vi "bazowy_TN_inz.vi"() -> ()   [LabVIEW 2019]
panel:
  out "komTESTz":bool
  out "komTESTdo":bool
  out "Objętość - zb4":dbl
  out "Objętość - zb3":dbl
  out "Objętość - zb2":dbl
  out "Objętość - zb1":dbl
  out "Zawór spustowy Z4":bool
  out "Zawór spustowy Z3":bool
  out "Zawór spustowy Z2":bool
  out "Zawór spustowy Z1":bool
  out "P8 - konserwacja":bool
  out "P7 - konserwacja":bool
  out "P6 - konserwacja":bool
  out "P5 - konserwacja":bool
  out "P4 - konserwacja":bool
  out "P3 - konserwacja":bool
  out "P2 - konserwacja":bool
  out "P1 - konserwacja":bool
  out "Awaryjne zatrzymanie pomp i opróżnienie  zbiorników (Awaria)":bool
  out "Czas utrzymania temperatury - zb4":u32
  out "Temperatura maksymalna - zb4":sgl
  out "Objętość cieczy - zb4":sgl
  out "Czas utrzymania temperatury - zb3":u32
  out "Temperatura maksymalna - zb3":sgl
  out "Objętość cieczy - zb3":sgl
  out "Czas utrzymania temperatury - zb2":u32
  out "Temperatura maksymalna - zb2":sgl
  out "Czas utrzymania temperatury - zb1":u32
  out "Objętość cieczy - zb2":sgl
  out "Temperatura maksymalna - zb1":sgl
  out "Objętość cieczy - zb1":sgl
  out "Grzałka 4":bool
  out "Grzałka 3":bool
  out "Grzałka 2":bool
  out "Grzałka 1":bool
  out "Pompa 8":bool
  out "Pompa 7":bool
  out "Pompa 6":bool
  out "Pompa 5":bool
  out "Pompa 4":bool
  out "Pompa 3":bool
  out "Pompa 2":bool
  out "Zawór wlotowy 3":bool
  out "Zawór wlotowy 2":bool
  out "Temp cieczy w zb 4":sgl
  out "Temp cieczy w zb 3":sgl
  out "Temp cieczy w zb 2":sgl
  out "Temp cieczy w zb 1":sgl
  out "Temp P8":sgl
  out "Temp P7":sgl
  out "Temp P6":sgl
  out "Temp P5":sgl
  out "Temp P4":sgl
  out "Temp P3":sgl
  out "Temp P2":sgl
  out "Temp P1":sgl=20.009169
  out "Pompa 1":bool
  out "Zawór wlotowy 1":bool
  out "Inf - temp przed zb3":dbl
  out "Inf - temp przed zb2":dbl
  out "Inf - temp przed zb1":dbl
  out "Inf - temp przed zb4":dbl
  out "Inf - poz przed zb3":dbl
  out "Inf - poz przed zb2":dbl
  out "Inf - poz przed zb1":dbl
  out "Temp. cieczy w zb 4":sgl
  out "Temp i objętość cieczy w zb 4":cluster{sgl, "T":dbl}(graph)
  out "Zbiornik 4":sgl(slide) scale=0.0..300.0
  out "Zbiornik 3":sgl(slide) scale=0.0..100.0
  out "Zbiornik 2":sgl(slide) scale=0.0..100.0
  out "Zbiornik 1":sgl(slide) scale=0.0..100.0
  out "Temp. cieczy w zb 3":sgl
  out "Temp. cieczy w zb 2":sgl
  out "Temp. cieczy w zb 1":sgl
  out "Temp i objętość cieczy w zb 3":cluster{"Zbiornik 3":sgl, "T":dbl}(graph)
  out "Temp i objętość cieczy w zb 2":cluster{"Zbiornik 2":sgl, "T":dbl}(graph)
  out "Temp i objętość cieczy w zb 1":cluster{"Zbiornik 1":sgl, "T":dbl}(graph)
  in  "r4d":sgl=0.002
  in  "r4":sgl=0.9977
  in  "r3d":sgl=0.02
  in  "r3":sgl=0.968
  in  "Tk":sgl=100.0
  in  "Tot":sgl=20.0
  out "Temp. P8":sgl
  out "Temp. P7":sgl
  out "temp P7 - P8":cluster{"T":dbl, "T":dbl, sgl}(graph)
  out "Temp. P6":sgl
  out "Temp. P5":sgl
  out "temp P5 - P6":cluster{"T":dbl, "T":dbl, "Zbiornik 3":sgl}(graph)
  out "Temp. P4":sgl
  out "Temp. P3":sgl
  out "temp P3 - P4":cluster{"T":dbl, "T":dbl, "Zbiornik 2":sgl}(graph)
  out "Temp. P2":sgl
  out "Temp. P1":sgl
  out "temp P1 - P2":cluster{"T":dbl, "T":dbl, "Zbiornik 1":sgl}(graph)
  in  "To":sgl=20.0
  in  "Ts":sgl=80.0
  in  "r2":sgl=0.92
  in  "r1":sgl=0.92
  in  "stop":bool
  # "Temperatura pomp"
  # "460 na wykres"
  # "(°C)"
  # "(°C)"
  # "(°C)"
  # "(°C)"
  # "(°C)"
  # "(°C)"
  # "(°C)"
  # "(°C)"
  # "(°C)"
  # "(°C)"
  # "Temperatura i objętość cieczy w zbiornikach 1, 2, 3 i 4"
  # "(°C)"
  # "(°C)"
  # "Nastawy grzanie"
  # "Nastawy chłodzenie"
  # "(°C)"
  # "(l)"
  # "(l)"
  # "(°C)"
  # "(°C)"
  # "(l)"
  # "(l)"
  # "(°C)"
  # "Nie do odczytu. Wartości chwilowe dla wyliczenia temperatury cieczy z zbiorników po zmieszaniu się"
  # "Parametry zadane w aktualnym procesie (partii produktu)"
  # "Zbiornik 1"
  # "Zbiornik 2"
  # "Zbiornik 3"
  # "(°C)"
  # "(°C)"
  # "(°C)"
  # "Zbiornik 4"
  # "(°C)"
  # "(°C)"
  # "(°C)"
  # "(°C)"
  # "(°C)"
  # "(°C)"
  # "(°C)"
  # "(°C)"
  # "(°C)"
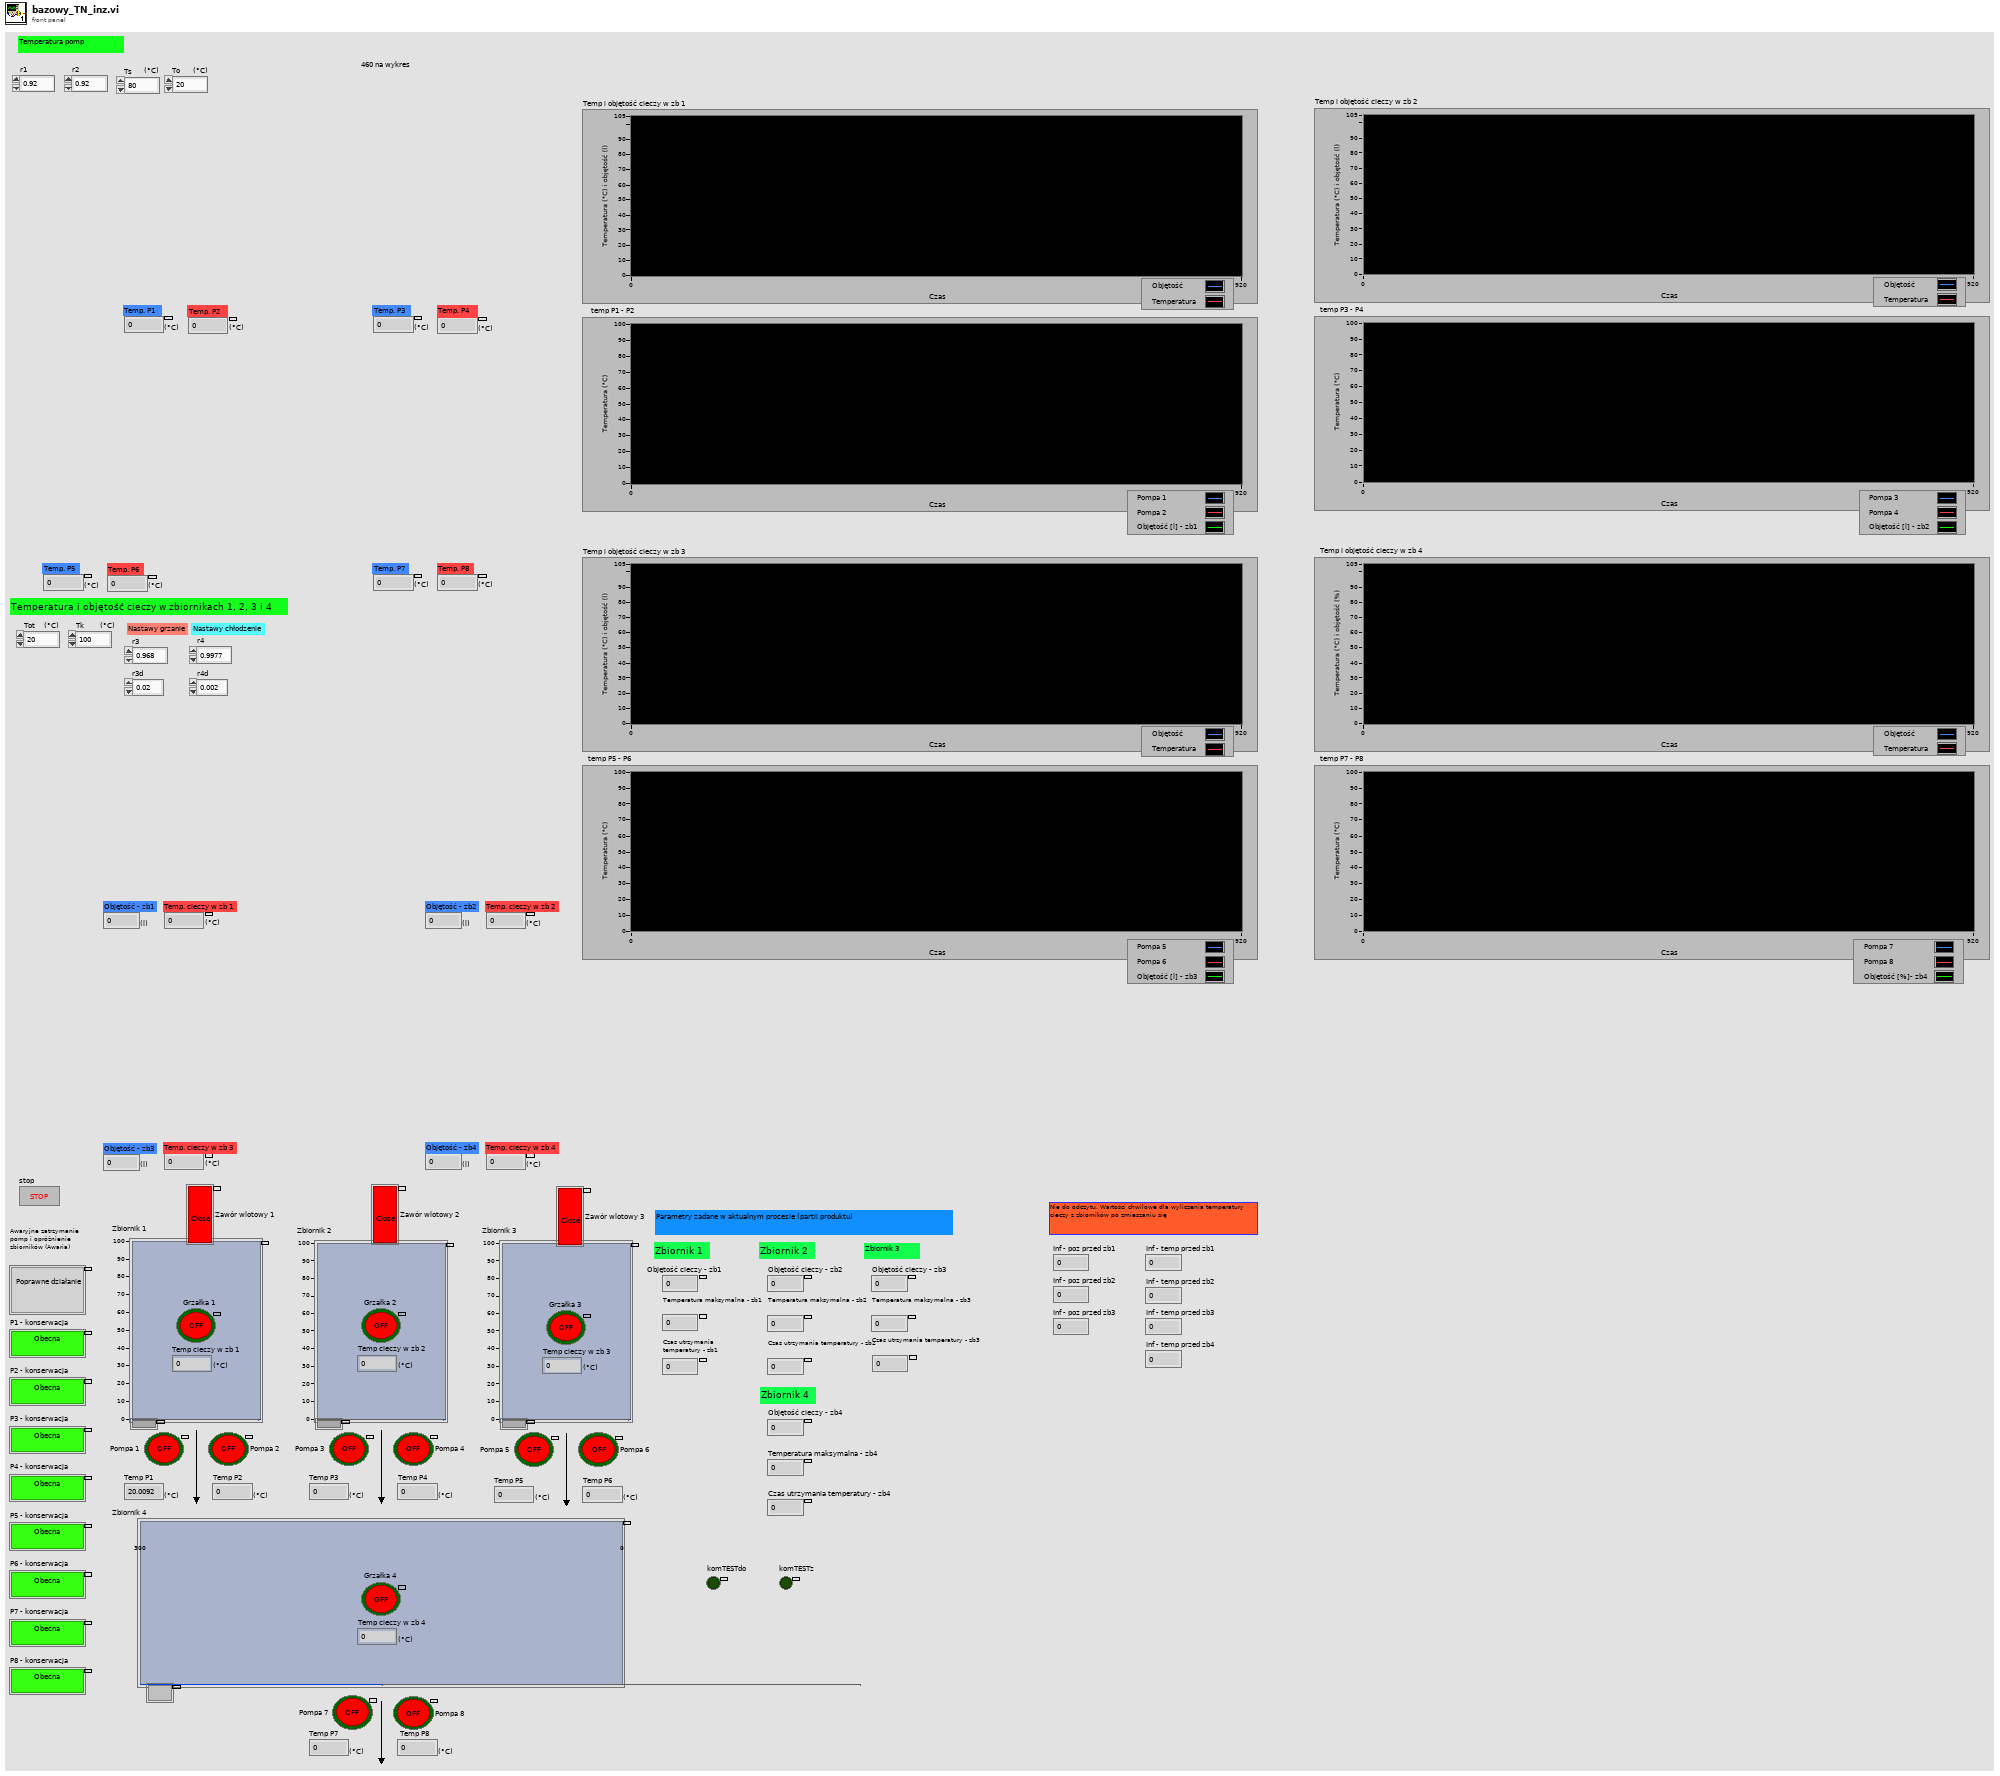
[diagram p1: front panel]
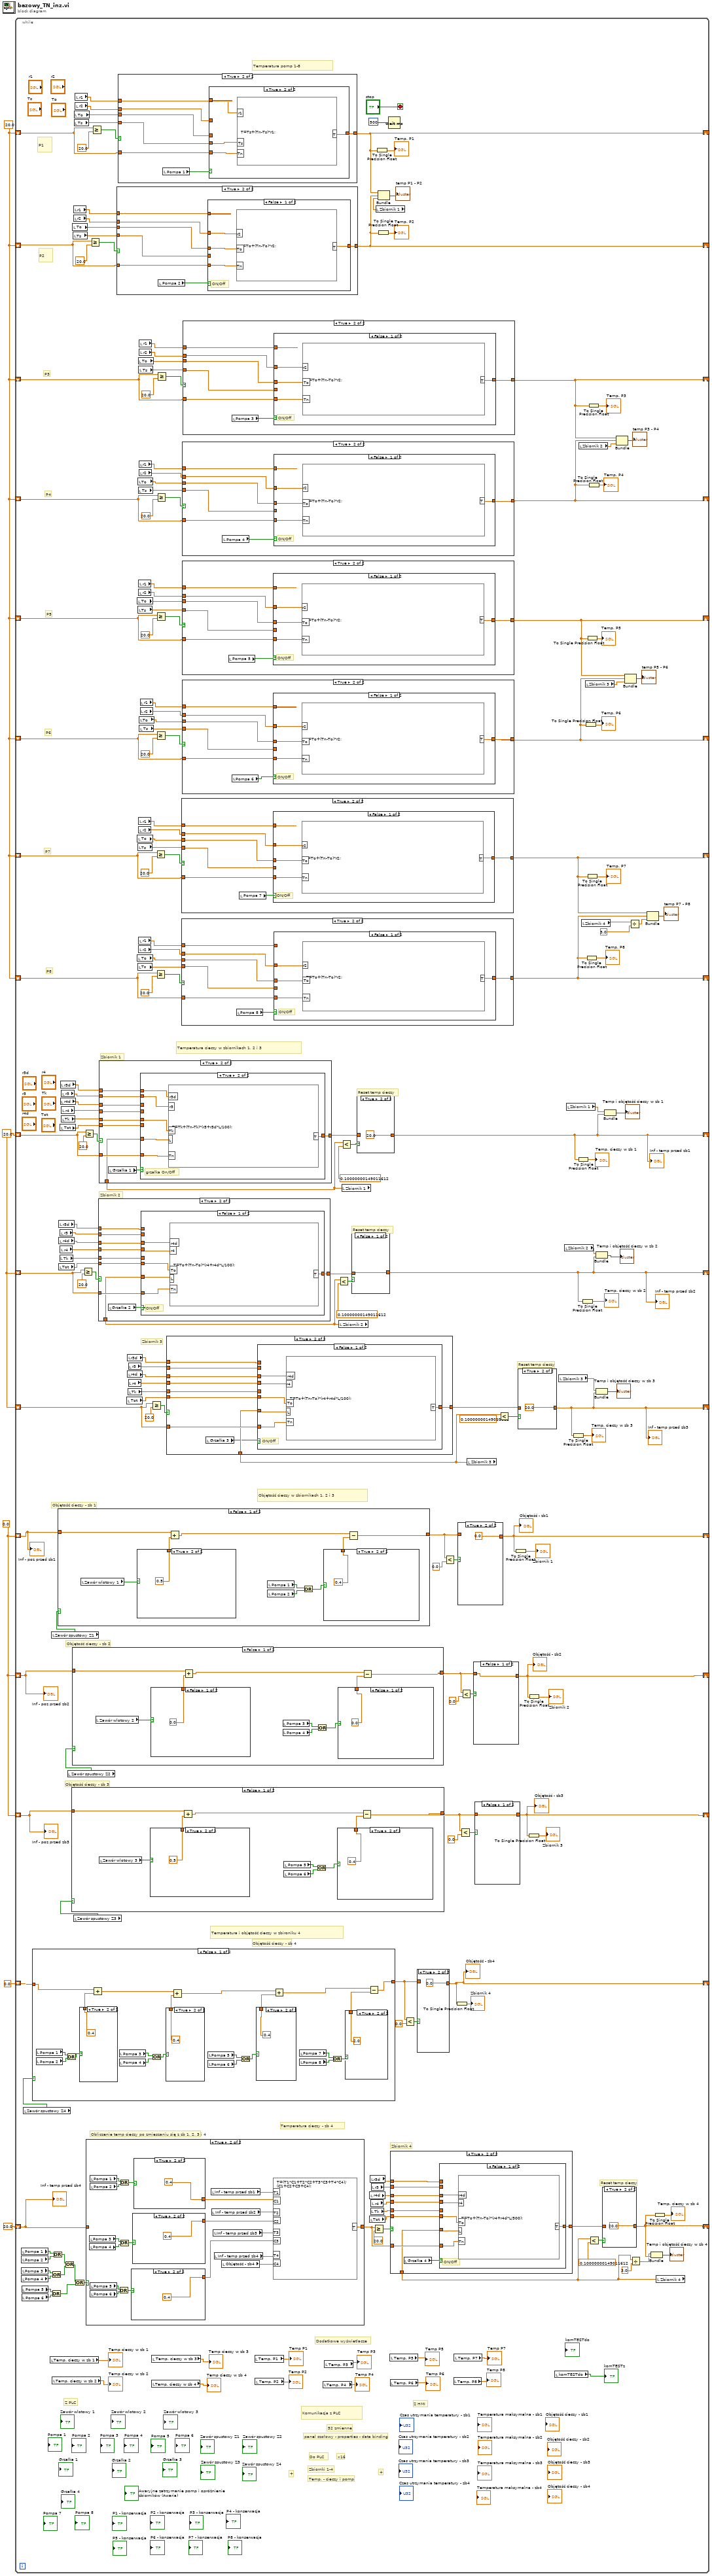
[diagram p0: block diagram]
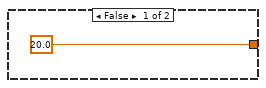
[diagram p2: hidden frame]
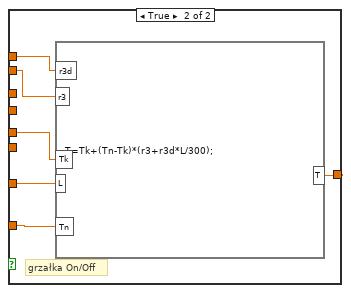
[diagram p3: hidden frame]
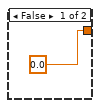
[diagram p5: hidden frame]
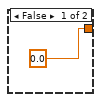
[diagram p6: hidden frame]
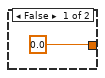
[diagram p7: hidden frame]
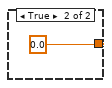
[diagram p9: hidden frame]
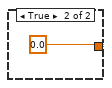
[diagram p10: hidden frame]
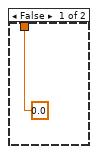
[diagram p12: hidden frame]
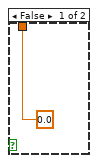
[diagram p13: hidden frame]
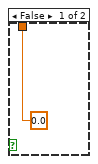
[diagram p14: hidden frame]
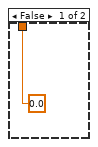
[diagram p15: hidden frame]
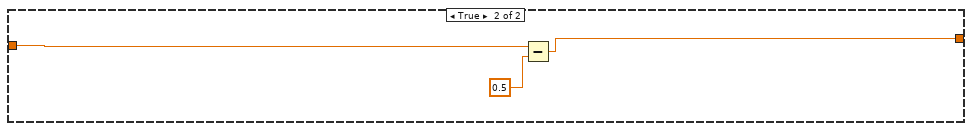
[diagram p16: hidden frame]
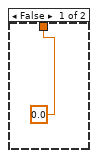
[diagram p18: hidden frame]
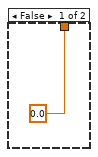
[diagram p19: hidden frame]
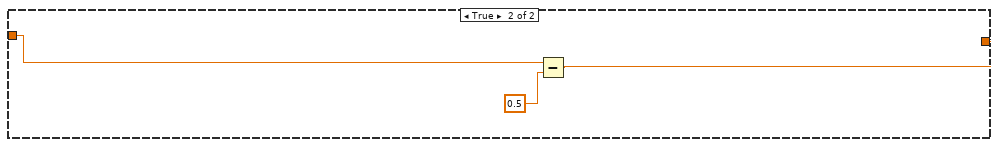
[diagram p20: hidden frame]
diagram:
  w4 = 0.0
  w1 = 20.0
  w5 = 20.0
  n1 = while {
    shift-right: [w60] -> _
    shift-left: w5 -> [w207]
    shift-right: [w59] -> _
    shift-left: w5 -> [w204]
    shift-right: [w58] -> _
    shift-left: w5 -> [w201]
    shift-right: [w57] -> _
    shift-left: w5 -> [w190]
    shift-right: [w53] -> _
    shift-left: w5 -> [w189]
    shift-right: [w55] -> _
    shift-left: w5 -> [w188]
    shift-right: [w52] -> _
    shift-left: w5 -> [w187]
    shift-right: [w54] -> _
    shift-left: w5 -> [w186]
    shift-right: [w16] -> _
    shift-left: w1 -> [w21]
    shift-right: [w15] -> _
    shift-left: w1 -> [w83]
    shift-right: [w14] -> _
    shift-left: w1 -> [w22]
    shift-right: [w37] -> _
    shift-left: w4 -> [w13]
    shift-right: [w39] -> _
    shift-left: w4 -> [w23]
    shift-right: [w38] -> _
    shift-left: w4 -> [w79]
    shift-right: [w41] -> _
    shift-left: 20.0 -> [w25]
    shift-right: [w40] -> _
    shift-left: 0.0 -> [w24]
    stop <- "stop" stop-if-true
    # "Temperatura cieczy - zb 4"
    # "x16"
    # "52 zmienne"
    # "Do PLC"
    # "Z PLC"
    # "Z HMI"
    # "panel czołowy - properties - data binding"
    # "Temp. - cieczy i pomp"
    # "Zbiornki 1-4"
    # "+"
    # "+"
    # "Dodatkowe wyświetlacze"
    # "Komunikacja z PLC"
    # "Obliczenie temp cieczy po zmieszaniu się z zb 1, 2, 3 i 4"
    # "Zbiornik 4"
    # "Reset temp cieczy"
    # "Objętość cieczy - zb 4"
    # "Temperatura i objętość cieczy w zbironiku 4"
    # "Objętość cieczy - zb 3"
    # "Objętość cieczy - zb 2"
    # "Objętość cieczy - zb 1"
    # "Objętość cieczy w zbiornikach 1, 2 i 3"
    # "Zbiornik 3"
    # "Reset temp cieczy"
    # "Zbiornik 2"
    # "Reset temp cieczy"
    # "Zbiornik 1"
    # "Reset temp cieczy"
    # "P8"
    # "P7"
    # "P6"
    # "P5"
    # "P4"
    # "Temperatura cieczy w zbiornikach 1, 2 i 3"
    # "P3"
    # "P2"
    # "P1"
    # "Temperatura pomp 1-8"
    n2 = local read "Pompa 1"() -> (w36:bool)
    n3 = local read "Pompa 2"() -> (w35:bool)
    n4 = local read "Pompa 3"() -> (w34:bool)
    n5 = local read "Pompa 4"() -> (w33:bool)
    n6 = local read "Pompa 5"() -> (w32:bool)
    n7 = local read "Pompa 6"() -> (w31:bool)
    n8 = local read "Zawór spustowy Z4"() -> (w95:bool)
    n9 = case shown="False" w95 {
      tunnel: [w284 w297] -> w118
      tunnel: w24 -> [w288 w298]
      frame False {
        n10 = local read "Pompa 1"() -> (w275:bool)
        n11 = local read "Pompa 2"() -> (w274:bool)
        n12 = Or(x=w275, y=w274) -> (x .or. y?=w280:bool)
        n13 = case shown="True" w280 {
          tunnel: [0.0 0.4] -> w279
          frame False {
          }
          frame True {
          }
        }
        n14 = Add(x=w288, y=w279) -> (x+y=w287:dbl)
        n15 = local read "Pompa 3"() -> (w273:bool)
        n16 = local read "Pompa 4"() -> (w272:bool)
        n17 = Or(x=w273, y=w272) -> (x .or. y?=w281:bool)
        n18 = case shown="True" w281 {
          tunnel: [0.0 0.4] -> w278
          frame False {
          }
          frame True {
          }
        }
        n19 = Add(x=w287, y=w278) -> (x+y=w286:dbl)
        n20 = local read "Pompa 5"() -> (w271:bool)
        n21 = local read "Pompa 6"() -> (w270:bool)
        n22 = Or(x=w271, y=w270) -> (x .or. y?=w282:bool)
        n23 = case shown="True" w282 {
          tunnel: [0.0 0.4] -> w277
          frame False {
          }
          frame True {
          }
        }
        n24 = Add(x=w286, y=w277) -> (x+y=w285:dbl)
        n25 = local read "Pompa 7"() -> (w269:bool)
        n26 = local read "Pompa 8"() -> (w268:bool)
        n27 = Or(x=w269, y=w268) -> (x .or. y?=w283:bool)
        n28 = case shown="True" w283 {
          tunnel: [0.0 2.0] -> w276
          frame False {
          }
          frame True {
          }
        }
        n29 = Subtract(x=w285, y=w276) -> (x-y=w284:dbl)
      }
      frame True {
        n30 = Subtract(x=w298, y=0.5) -> (x-y=w297:dbl)
      }
    }
    n31 = local read "Temp. cieczy w zb 1"() -> (→"Temp cieczy w zb 1":sgl)
    n32 = Or(x=w32, y=w31) -> (x .or. y?=w28:bool)
    n33 = Or(x=w34, y=w33) -> (x .or. y?=w29:bool)
    n34 = local read "Zawór spustowy Z1"() -> (w93:bool)
    n35 = Or(x=w36, y=w35) -> (x .or. y?=w30:bool)
    n36 = local read "Temp. cieczy w zb 2"() -> (→"Temp cieczy w zb 2":sgl)
    n37 = case shown="False" w93 {
      tunnel: w13 -> [w342 w349]
      tunnel: [w340 w347] -> w127
      frame False {
        n38 = local read "Zawór wlotowy 1"() -> (w336:bool)
        n39 = case shown="True" w336 {
          tunnel: [0.0 0.5] -> w338
          frame False {
          }
          frame True {
          }
        }
        n40 = Add(x=w342, y=w338) -> (x+y=w341:dbl)
        n41 = local read "Pompa 1"() -> (w335:bool)
        n42 = local read "Pompa 2"() -> (w334:bool)
        n43 = Or(x=w335, y=w334) -> (x .or. y?=w339:bool)
        n44 = case shown="True" w339 {
          tunnel: [0.0 0.4] -> w337
          frame False {
          }
          frame True {
          }
        }
        n45 = Subtract(x=w341, y=w337) -> (x-y=w340:dbl)
      }
      frame True {
        n46 = Subtract(x=w349, y=0.5) -> (x-y=w347:dbl)
      }
    }
    n47 = local read "Tot"() -> (w136:sgl)
    n48 = local read "r3d"() -> (w141:sgl)
    n49 = local read "r4d"() -> (w139:sgl)
    n50 = local read "Tk"() -> (w137:sgl)
    n51 = local read "Tot"() -> (w142:sgl)
    n52 = local read "r3"() -> (w140:sgl)
    n53 = local read "r4"() -> (w138:sgl)
    n54 = local read "r3d"() -> (w147:sgl)
    n55 = local read "r4d"() -> (w145:sgl)
    n56 = local read "Tk"() -> (w143:sgl)
    n57 = local read "r3"() -> (w146:sgl)
    n58 = local read "r4"() -> (w144:sgl)
    n59 = Or(x=w30, y=w29) -> (x .or. y?=w27:bool)
    n60 = local read "Zawór spustowy Z2"() -> (w92:bool)
    n61 = case shown="False" w92 {
      tunnel: w79 -> [w326 w333]
      tunnel: [w324 w331] -> w121
      frame False {
        n62 = local read "Zawór wlotowy 2"() -> (w320:bool)
        n63 = case shown="False" w320 {
          tunnel: [0.0 0.5] -> w322
          frame False {
          }
          frame True {
          }
        }
        n64 = Add(x=w326, y=w322) -> (x+y=w325:dbl)
        n65 = local read "Pompa 3"() -> (w319:bool)
        n66 = local read "Pompa 4"() -> (w318:bool)
        n67 = Or(x=w319, y=w318) -> (x .or. y?=w323:bool)
        n68 = case shown="False" w323 {
          tunnel: [0.0 0.4] -> w321
          frame False {
          }
          frame True {
          }
        }
        n69 = Subtract(x=w325, y=w321) -> (x-y=w324:dbl)
      }
      frame True {
        n70 = Subtract(x=w333, y=0.5) -> (x-y=w331:dbl)
      }
    }
    n71 = local read "To"() -> (w153:sgl)
    n72 = local read "Ts"() -> (w152:sgl)
    n73 = local read "r1"() -> (w155:sgl)
    n74 = local read "r2"() -> (w154:sgl)
    n75 = local read "Zawór spustowy Z3"() -> (w94:bool)
    n76 = case shown="False" w94 {
      tunnel: w23 -> [w310 w317]
      tunnel: [w308 w316] -> w122
      frame False {
        n77 = local read "Zawór wlotowy 3"() -> (w304:bool)
        n78 = case shown="True" w304 {
          tunnel: [0.0 0.5] -> w306
          frame False {
          }
          frame True {
          }
        }
        n79 = Add(x=w310, y=w306) -> (x+y=w309:dbl)
        n80 = local read "Pompa 5"() -> (w303:bool)
        n81 = local read "Pompa 6"() -> (w302:bool)
        n82 = Or(x=w303, y=w302) -> (x .or. y?=w307:bool)
        n83 = case shown="True" w307 {
          tunnel: [0.0 0.4] -> w305
          frame False {
          }
          frame True {
          }
        }
        n84 = Subtract(x=w309, y=w305) -> (x-y=w308:dbl)
      }
      frame True {
        n85 = Subtract(x=w317, y=0.5) -> (x-y=w316:dbl)
      }
    }
    n86 = local read "To"() -> (w157:sgl)
    n87 = local read "Ts"() -> (w156:sgl)
    n88 = Or(x=w27, y=w28) -> (x .or. y?=w26:bool)
    n89 = local read "r1"() -> (w159:sgl)
    n90 = local read "r2"() -> (w158:sgl)
    n91 = Greater Or Equal?(x=w83, y=20.0) -> (x >= y?=w183:bool)
    n92 = Greater Or Equal?(x=w21, y=20.0) -> (x >= y?=w185:bool)
    n93 = case shown="True" w26 {
      tunnel: [w235 w253] -> w115
      tunnel: w25 -> [w235 _]
      frame False {
      }
      frame True {
        n94 = local read "Pompa 3"() -> (w250:bool)
        n95 = local read "Pompa 4"() -> (w249:bool)
        n96 = local read "Pompa 1"() -> (w252:bool)
        n97 = local read "Pompa 2"() -> (w251:bool)
        n98 = local read "Pompa 5"() -> (w248:bool)
        n99 = local read "Pompa 6"() -> (w247:bool)
        n100 = Or(x=w248, y=w247) -> (x .or. y?=w244:bool)
        n101 = Or(x=w252, y=w251) -> (x .or. y?=w246:bool)
        n102 = Or(x=w250, y=w249) -> (x .or. y?=w245:bool)
        n103 = case shown="True" w244 {
          tunnel: [0.0 0.4] -> w243
          frame False {
          }
          frame True {
          }
        }
        n104 = case shown="True" w245 {
          tunnel: [0.0 0.4] -> w241
          frame False {
          }
          frame True {
          }
        }
        n105 = case shown="True" w246 {
          tunnel: [0.0 0.4] -> w242
          frame False {
          }
          frame True {
          }
        }
        n106 = local read "Inf - temp przed zb1"() -> (w238:dbl)
        n107 = local read "Inf - temp przed zb2"() -> (w237:dbl)
        n108 = local read "Inf - temp przed zb3"() -> (w236:dbl)
        n109 = local read "Inf - temp przed zb4"() -> (w240:dbl)
        n110 = local read "Objętość - zb4"() -> (w239:dbl)
        n111 = formula code="T=(T1*C1+T2*C2+T3*C3+T4*C4)/\n(C1+C2+C3+C4);"("T1"=w238, "C1"=w242, "T2"=w237, "C2"=w241, "T3"=w236, "C3"=w243, "T4"=w240, "C4"=w239) -> ("T"=w253:dbl)
      }
    }
    n112 = Greater Or Equal?(x=w204, y=20.0) -> (x >= y?=w206:bool)
    n113 = Greater Or Equal?(x=w207, y=20.0) -> (x >= y?=w209:bool)
    n114 = case shown="True" w206 {
      tunnel: w204 -> [_ w528]
      tunnel: [20.0 w527] -> w59
      tunnel: w155 -> [_ w526]
      tunnel: w154 -> [_ w525]
      tunnel: w152 -> [_ w524]
      tunnel: w153 -> [_ w523]
      frame False {
      }
      frame True {
        n115 = local read "Pompa 2"() -> (w522:bool)
        n116 = case shown="False" w522 {
          tunnel: w528 -> [w529 w536]
          tunnel: [w532 w533] -> w527
          tunnel: w526 -> [_ w535]
          tunnel: w525 -> [w531 _]
          tunnel: w524 -> [_ w534]
          tunnel: w523 -> [w530 _]
          frame False {
            # "ON/Off"
            n117 = formula code="T=To+(Tn-To)*r2;"("r2"=w531, "To"=w530, "Tn"=w529) -> ("T"=w532:dbl)
          }
          frame True {
            n118 = formula code="T=Ts+(Tn-Ts)*r1;"("r1"=w535, "Ts"=w534, "Tn"=w536) -> ("T"=w533:dbl)
          }
        }
      }
    }
    n119 = case shown="True" w209 {
      tunnel: w207 -> [_ w544]
      tunnel: [20.0 w543] -> w60
      tunnel: w159 -> [_ w542]
      tunnel: w158 -> [_ w541]
      tunnel: w156 -> [_ w540]
      tunnel: w157 -> [_ w539]
      frame False {
      }
      frame True {
        n120 = local read "Pompa 1"() -> (w538:bool)
        n121 = case shown="True" w538 {
          tunnel: w544 -> [w545 w552]
          tunnel: [w548 w549] -> w543
          tunnel: w542 -> [_ w551]
          tunnel: w541 -> [w547 _]
          tunnel: w540 -> [_ w550]
          tunnel: w539 -> [w546 _]
          frame False {
            # "ON/Off"
            n122 = formula code="T=To+(Tn-To)*r2;"("r2"=w547, "To"=w546, "Tn"=w545) -> ("T"=w548:dbl)
          }
          frame True {
            n123 = formula code="T=Ts+(Tn-Ts)*r1;"("r1"=w551, "Ts"=w550, "Tn"=w552) -> ("T"=w549:dbl)
          }
        }
      }
    }
    n124 = local read "Tot"() -> (w130:sgl)
    n125 = local read "r3d"() -> (w135:sgl)
    n126 = local read "r4d"() -> (w133:sgl)
    n127 = local read "Tk"() -> (w131:sgl)
    n128 = local read "r3"() -> (w134:sgl)
    n129 = local read "r4"() -> (w132:sgl)
    n130 = local read "To"() -> (w166:sgl)
    n131 = local read "To"() -> (w173:sgl)
    n132 = local read "To"() -> (w178:sgl)
    n133 = local read "To"() -> (w162:sgl)
    n134 = local read "Ts"() -> (w167:sgl)
    n135 = local read "Ts"() -> (w172:sgl)
    n136 = local read "Ts"() -> (w179:sgl)
    n137 = local read "To"() -> (w149:sgl)
    n138 = local read "Ts"() -> (w163:sgl)
    n139 = local read "Ts"() -> (w148:sgl)
    n140 = local read "r1"() -> (w164:sgl)
    n141 = local read "r2"() -> (w165:sgl)
    n142 = local read "r1"() -> (w175:sgl)
    n143 = local read "r2"() -> (w174:sgl)
    n144 = local read "r1"() -> (w176:sgl)
    n145 = local read "r2"() -> (w177:sgl)
    n146 = local read "r1"() -> (w160:sgl)
    n147 = local read "r2"() -> (w161:sgl)
    n148 = local read "To"() -> (w170:sgl)
    n149 = local read "r1"() -> (w151:sgl)
    n150 = local read "r2"() -> (w150:sgl)
    n151 = local read "Ts"() -> (w171:sgl)
    n152 = local read "r1"() -> (w168:sgl)
    n153 = local read "r2"() -> (w169:sgl)
    n154 = Greater Or Equal?(x=w22, y=20.0) -> (x >= y?=w181:bool)
    n155 = local read "Temp. cieczy w zb 4"() -> (→"Temp cieczy w zb 4":sgl)
    n156 = local read "Temp. cieczy w zb 3"() -> (→"Temp cieczy w zb 3":sgl)
    n157 = Greater Or Equal?(x=w187, y=20.0) -> (x >= y?=w194:bool)
    n158 = Greater Or Equal?(x=w186, y=20.0) -> (x >= y?=w192:bool)
    n159 = Greater Or Equal?(x=w189, y=20.0) -> (x >= y?=w198:bool)
    n160 = Greater Or Equal?(x=w188, y=20.0) -> (x >= y?=w196:bool)
    n161 = Greater Or Equal?(x=w190, y=20.0) -> (x >= y?=w200:bool)
    n162 = Greater Or Equal?(x=w201, y=20.0) -> (x >= y?=w203:bool)
    n163 = case shown="True" w194 {
      tunnel: w187 -> [_ w448]
      tunnel: [20.0 w447] -> w52
      tunnel: w175 -> [_ w446]
      tunnel: w174 -> [_ w445]
      tunnel: w172 -> [_ w444]
      tunnel: w173 -> [_ w443]
      frame False {
      }
      frame True {
        n164 = local read "Pompa 7"() -> (w442:bool)
        n165 = case shown="False" w442 {
          tunnel: w448 -> [w449 w456]
          tunnel: [w452 w453] -> w447
          tunnel: w446 -> [_ w455]
          tunnel: w445 -> [w451 _]
          tunnel: w444 -> [_ w454]
          tunnel: w443 -> [w450 _]
          frame False {
            # "ON/Off"
            n166 = formula code="T=To+(Tn-To)*r2;"("r2"=w451, "To"=w450, "Tn"=w449) -> ("T"=w452:dbl)
          }
          frame True {
            n167 = formula code="T=Ts+(Tn-Ts)*r1;"("r1"=w455, "Ts"=w454, "Tn"=w456) -> ("T"=w453:dbl)
          }
        }
      }
    }
    n168 = case shown="True" w192 {
      tunnel: w186 -> [_ w432]
      tunnel: [20.0 w431] -> w54
      tunnel: w176 -> [_ w430]
      tunnel: w177 -> [_ w429]
      tunnel: w179 -> [_ w428]
      tunnel: w178 -> [_ w427]
      frame False {
      }
      frame True {
        n169 = local read "Pompa 8"() -> (w426:bool)
        n170 = case shown="False" w426 {
          tunnel: w432 -> [w433 w440]
          tunnel: [w436 w437] -> w431
          tunnel: w430 -> [_ w439]
          tunnel: w429 -> [w435 _]
          tunnel: w428 -> [_ w438]
          tunnel: w427 -> [w434 _]
          frame False {
            # "ON/Off"
            n171 = formula code="T=To+(Tn-To)*r2;"("r2"=w435, "To"=w434, "Tn"=w433) -> ("T"=w436:dbl)
          }
          frame True {
            n172 = formula code="T=Ts+(Tn-Ts)*r1;"("r1"=w439, "Ts"=w438, "Tn"=w440) -> ("T"=w437:dbl)
          }
        }
      }
    }
    n173 = case shown="True" w198 {
      tunnel: w189 -> [_ w480]
      tunnel: [20.0 w479] -> w53
      tunnel: w164 -> [_ w478]
      tunnel: w165 -> [_ w477]
      tunnel: w167 -> [_ w476]
      tunnel: w166 -> [_ w475]
      frame False {
      }
      frame True {
        n174 = local read "Pompa 5"() -> (w474:bool)
        n175 = case shown="False" w474 {
          tunnel: w480 -> [w481 w488]
          tunnel: [w484 w485] -> w479
          tunnel: w478 -> [_ w487]
          tunnel: w477 -> [w483 _]
          tunnel: w476 -> [_ w486]
          tunnel: w475 -> [w482 _]
          frame False {
            # "ON/Off"
            n176 = formula code="T=To+(Tn-To)*r2;"("r2"=w483, "To"=w482, "Tn"=w481) -> ("T"=w484:dbl)
          }
          frame True {
            n177 = formula code="T=Ts+(Tn-Ts)*r1;"("r1"=w487, "Ts"=w486, "Tn"=w488) -> ("T"=w485:dbl)
          }
        }
      }
    }
    n178 = case shown="True" w196 {
      tunnel: w188 -> [_ w464]
      tunnel: [20.0 w463] -> w55
      tunnel: w168 -> [_ w462]
      tunnel: w169 -> [_ w461]
      tunnel: w171 -> [_ w460]
      tunnel: w170 -> [_ w459]
      frame False {
      }
      frame True {
        n179 = local read "Pompa 6"() -> (w458:bool)
        n180 = case shown="False" w458 {
          tunnel: w464 -> [w465 w472]
          tunnel: [w468 w469] -> w463
          tunnel: w462 -> [_ w471]
          tunnel: w461 -> [w467 _]
          tunnel: w460 -> [_ w470]
          tunnel: w459 -> [w466 _]
          frame False {
            # "ON/Off"
            n181 = formula code="T=To+(Tn-To)*r2;"("r2"=w467, "To"=w466, "Tn"=w465) -> ("T"=w468:dbl)
          }
          frame True {
            n182 = formula code="T=Ts+(Tn-Ts)*r1;"("r1"=w471, "Ts"=w470, "Tn"=w472) -> ("T"=w469:dbl)
          }
        }
      }
    }
    n183 = case shown="True" w200 {
      tunnel: w190 -> [_ w496]
      tunnel: [20.0 w495] -> w57
      tunnel: w160 -> [_ w494]
      tunnel: w161 -> [_ w493]
      tunnel: w163 -> [_ w492]
      tunnel: w162 -> [_ w491]
      frame False {
      }
      frame True {
        n184 = local read "Pompa 4"() -> (w490:bool)
        n185 = case shown="False" w490 {
          tunnel: w496 -> [w497 w504]
          tunnel: [w500 w501] -> w495
          tunnel: w494 -> [_ w503]
          tunnel: w493 -> [w499 _]
          tunnel: w492 -> [_ w502]
          tunnel: w491 -> [w498 _]
          frame False {
            # "ON/Off"
            n186 = formula code="T=To+(Tn-To)*r2;"("r2"=w499, "To"=w498, "Tn"=w497) -> ("T"=w500:dbl)
          }
          frame True {
            n187 = formula code="T=Ts+(Tn-Ts)*r1;"("r1"=w503, "Ts"=w502, "Tn"=w504) -> ("T"=w501:dbl)
          }
        }
      }
    }
    n188 = case shown="True" w203 {
      tunnel: w201 -> [_ w512]
      tunnel: [20.0 w511] -> w58
      tunnel: w151 -> [_ w510]
      tunnel: w150 -> [_ w509]
      tunnel: w148 -> [_ w508]
      tunnel: w149 -> [_ w507]
      frame False {
      }
      frame True {
        n189 = local read "Pompa 3"() -> (w506:bool)
        n190 = case shown="False" w506 {
          tunnel: w512 -> [w513 w520]
          tunnel: [w516 w517] -> w511
          tunnel: w510 -> [_ w519]
          tunnel: w509 -> [w515 _]
          tunnel: w508 -> [_ w518]
          tunnel: w507 -> [w514 _]
          frame False {
            # "ON/Off"
            n191 = formula code="T=To+(Tn-To)*r2;"("r2"=w515, "To"=w514, "Tn"=w513) -> ("T"=w516:dbl)
          }
          frame True {
            n192 = formula code="T=Ts+(Tn-Ts)*r1;"("r1"=w519, "Ts"=w518, "Tn"=w520) -> ("T"=w517:dbl)
          }
        }
      }
    }
    n193 = local read "Temp. P1"() -> (→"Temp P1":sgl)
    n194 = local read "Temp. P2"() -> (→"Temp P2":sgl)
    n195 = local read "Temp. P4"() -> (→"Temp P4":sgl)
    n196 = local read "Temp. P3"() -> (→"Temp P3":sgl)
    n197 = local read "Zbiornik 2"() -> (w67:sgl)
    n198 = case shown="True" w183 {
      tunnel: w83 -> [_ w387]
      tunnel: [20.0 w386] -> w50
      tunnel: w136 -> [_ w385]
      tunnel: w137 -> [_ w384]
      tunnel: w138 -> [_ w383]
      tunnel: w139 -> [_ w382]
      tunnel: w140 -> [_ w381]
      tunnel: w141 -> [_ w380]
      tunnel: w67 -> [_ w379]
      frame False {
      }
      frame True {
        n199 = local read "Grzałka 2"() -> (w378:bool)
        n200 = case shown="False" w378 {
          tunnel: w387 -> [w392 w399]
          tunnel: [w393 w398] -> w386
          tunnel: w385 -> [w389 _]
          tunnel: w384 -> [_ w395]
          tunnel: w383 -> [w390 _]
          tunnel: w382 -> [w391 _]
          tunnel: w381 -> [_ w396]
          tunnel: w380 -> [_ w397]
          tunnel: w379 -> [w388 w394]
          frame False {
            # "ON/Off"
            n201 = formula code="T=To+(Tn-To)*(r4+r4d*L/100);"("r4"=w390, "r4d"=w391, "To"=w389, "L"=w388, "Tn"=w392) -> ("T"=w393:dbl)
          }
          frame True {
            # "grzałka On/Off"
            n202 = formula code="T=Tk+(Tn-Tk)*(r3+r3d*L/100);"("r3"=w396, "r3d"=w397, "L"=w394, "Tk"=w395, "Tn"=w399) -> ("T"=w398:dbl)
          }
        }
      }
    }
    n203 = Less?(x=w67, y=sgl 0.1) -> (x < y?=w66:bool)
    n204 = local read "Zbiornik 1"() -> (w65:sgl)
    n205 = case shown="True" w185 {
      tunnel: w21 -> [_ w412]
      tunnel: [20.0 w411] -> w51
      tunnel: w142 -> [_ w410]
      tunnel: w143 -> [_ w409]
      tunnel: w144 -> [_ w408]
      tunnel: w145 -> [_ w407]
      tunnel: w146 -> [_ w406]
      tunnel: w147 -> [_ w405]
      tunnel: w65 -> [_ w404]
      frame False {
      }
      frame True {
        n206 = local read "Grzałka 1"() -> (w403:bool)
        n207 = case shown="True" w403 {
          tunnel: w412 -> [w417 w424]
          tunnel: [w418 w423] -> w411
          tunnel: w410 -> [w414 _]
          tunnel: w409 -> [_ w420]
          tunnel: w408 -> [w415 _]
          tunnel: w407 -> [w416 _]
          tunnel: w406 -> [_ w421]
          tunnel: w405 -> [_ w422]
          tunnel: w404 -> [w413 w419]
          frame False {
            # "grzałka ON/Off"
            n208 = formula code="T=To+(Tn-To)*(r4+r4d*L/100);"("r4"=w415, "r4d"=w416, "To"=w414, "L"=w413, "Tn"=w417) -> ("T"=w418:dbl)
          }
          frame True {
            # "grzałka On/Off"
            n209 = formula code="T=Tk+(Tn-Tk)*(r3+r3d*L/100);"("r3"=w421, "r3d"=w422, "L"=w419, "Tk"=w420, "Tn"=w424) -> ("T"=w423:dbl)
          }
        }
      }
    }
    n210 = Less?(x=w65, y=sgl 0.1) -> (x < y?=w64:bool)
    n211 = case shown="False" w66 {
      tunnel: [w375 20.0] -> w15
      tunnel: w50 -> [w375 _]
      frame False {
      }
      frame True {
      }
    }
    "Inf - temp przed zb2" <- w15
    n212 = case shown="True" w64 {
      tunnel: [w400 20.0] -> w16
      tunnel: w51 -> [w400 _]
      frame False {
      }
      frame True {
      }
    }
    "Inf - temp przed zb1" <- w16
    n213 = local read "Tot"() -> (w109:sgl)
    n214 = local read "r4d"() -> (w112:sgl)
    n215 = local read "r3d"() -> (w114:sgl)
    n216 = local read "Tk"() -> (w110:sgl)
    n217 = local read "r4"() -> (w111:sgl)
    n218 = local read "r3"() -> (w113:sgl)
    n219 = Greater Or Equal?(x=w115, y=20.0) -> (x >= y?=w117:bool)
    n220 = local read "Zbiornik 1"() -> (w12:sgl)
    n221 = To Single Precision Float(number=w60) -> (single precision float=→"Temp. P1":sgl)
    n222 = To Single Precision Float(number=w59) -> (single precision float=→"Temp. P2":sgl)
    n223 = Bundle("T"=w60, "T"=w59, "Zbiornik 1"=w12) -> (→"temp P1 - P2":cluster{"T":dbl, "T":dbl, "Zbiornik 1":sgl})  [unwired: 1 in]
    n224 = Wait (ms)(milliseconds to wait=u32 500) -> ()  [unwired: 1 out]
    n225 = local read "Temp. P5"() -> (→"Temp P5":sgl)
    n226 = local read "Temp. P6"() -> (→"Temp P6":sgl)
    n227 = Less?(x=w118, y=0.0) -> (x < y?=w120:bool)
    n228 = case shown="True" w120 {
      tunnel: [w260 0.0] -> w40
      tunnel: w118 -> [w260 _]
      frame False {
      }
      frame True {
      }
    }
    "Objętość - zb4" <- w40
    n229 = Less?(x=w127, y=0.0) -> (x < y?=w129:bool)
    n230 = local read "Temp. P8"() -> (→"Temp P8":sgl)
    n231 = local read "Temp. P7"() -> (→"Temp P7":sgl)
    n232 = To Single Precision Float(number=w40) -> (single precision float=→"Zbiornik 4":sgl)
    n233 = case shown="True" w129 {
      tunnel: [w266 0.0] -> w37
      tunnel: w127 -> [w266 _]
      frame False {
      }
      frame True {
      }
    }
    "Objętość - zb1" <- w37
    n234 = Less?(x=w122, y=0.0) -> (x < y?=w124:bool)
    n235 = Less?(x=w121, y=0.0) -> (x < y?=w126:bool)
    n236 = local read "Zbiornik 3"() -> (w69:sgl)
    n237 = case shown="True" w181 {
      tunnel: w22 -> [_ w362]
      tunnel: [20.0 w361] -> w49
      tunnel: w130 -> [_ w360]
      tunnel: w131 -> [_ w359]
      tunnel: w132 -> [_ w358]
      tunnel: w133 -> [_ w357]
      tunnel: w134 -> [_ w356]
      tunnel: w135 -> [_ w355]
      tunnel: w69 -> [_ w354]
      frame False {
      }
      frame True {
        n238 = local read "Grzałka 3"() -> (w353:bool)
        n239 = case shown="False" w353 {
          tunnel: w362 -> [w367 w374]
          tunnel: [w368 w373] -> w361
          tunnel: w360 -> [w364 _]
          tunnel: w359 -> [_ w370]
          tunnel: w358 -> [w365 _]
          tunnel: w357 -> [w366 _]
          tunnel: w356 -> [_ w371]
          tunnel: w355 -> [_ w372]
          tunnel: w354 -> [w363 w369]
          frame False {
            # "ON/Off"
            n240 = formula code="T=To+(Tn-To)*(r4+r4d*L/100);"("r4"=w365, "r4d"=w366, "To"=w364, "L"=w363, "Tn"=w367) -> ("T"=w368:dbl)
          }
          frame True {
            # "grzałka On/Off"
            n241 = formula code="T=Tk+(Tn-Tk)*(r3+r3d*L/100);"("r3"=w371, "r3d"=w372, "L"=w369, "Tk"=w370, "Tn"=w374) -> ("T"=w373:dbl)
          }
        }
      }
    }
    n242 = case shown="False" w126 {
      tunnel: [w264 0.0] -> w38
      tunnel: w121 -> [w264 _]
      frame False {
      }
      frame True {
      }
    }
    "Objętość - zb2" <- w38
    n243 = case shown="False" w124 {
      tunnel: [w262 0.0] -> w39
      tunnel: w122 -> [w262 _]
      frame False {
      }
      frame True {
      }
    }
    "Objętość - zb3" <- w39
    n244 = Less?(x=w69, y=sgl 0.1) -> (x < y?=w68:bool)
    n245 = To Single Precision Float(number=w37) -> (single precision float=→"Zbiornik 1":sgl)
    n246 = case shown="True" w68 {
      tunnel: [w350 20.0] -> w14
      tunnel: w49 -> [w350 _]
      frame False {
      }
      frame True {
      }
    }
    "Inf - temp przed zb3" <- w14
    n247 = To Single Precision Float(number=w39) -> (single precision float=→"Zbiornik 3":sgl)
    n248 = To Single Precision Float(number=w38) -> (single precision float=→"Zbiornik 2":sgl)
    n249 = local read "komTESTdo"() -> (→"komTESTz":bool)
    n250 = local read "Zbiornik 3"() -> (w42:sgl)
    n251 = local read "Zbiornik 2"() -> (w44:sgl)
    n252 = local read "Zbiornik 1"() -> (w47:sgl)
    n253 = To Single Precision Float(number=w14) -> (single precision float=→"Temp. cieczy w zb 3":sgl)
    n254 = To Single Precision Float(number=w16) -> (single precision float=→"Temp. cieczy w zb 1":sgl)
    n255 = local read "Zbiornik 2"() -> (w11:sgl)
    n256 = local read "Zbiornik 4"() -> (w7:sgl)
    n257 = To Single Precision Float(number=w15) -> (single precision float=→"Temp. cieczy w zb 2":sgl)
    n258 = To Single Precision Float(number=w55) -> (single precision float=→"Temp. P6":sgl)
    n259 = local read "Zbiornik 3"() -> (w10:sgl)
    n260 = To Single Precision Float(number=w54) -> (single precision float=→"Temp. P8":sgl)
    n261 = To Single Precision Float(number=w53) -> (single precision float=→"Temp. P5":sgl)
    n262 = To Single Precision Float(number=w52) -> (single precision float=→"Temp. P7":sgl)
    n263 = To Single Precision Float(number=w58) -> (single precision float=→"Temp. P3":sgl)
    n264 = To Single Precision Float(number=w57) -> (single precision float=→"Temp. P4":sgl)
    n265 = Bundle("Zbiornik 3"=w42, "T"=w14) -> (→"Temp i objętość cieczy w zb 3":cluster{"Zbiornik 3":sgl, "T":dbl})  [unwired: 1 in]
    n266 = Bundle("Zbiornik 2"=w44, "T"=w15) -> (→"Temp i objętość cieczy w zb 2":cluster{"Zbiornik 2":sgl, "T":dbl})  [unwired: 1 in]
    n267 = Bundle("Zbiornik 1"=w47, "T"=w16) -> (→"Temp i objętość cieczy w zb 1":cluster{"Zbiornik 1":sgl, "T":dbl})  [unwired: 1 in]
    n268 = Bundle("T"=w58, "T"=w57, "Zbiornik 2"=w11) -> (→"temp P3 - P4":cluster{"T":dbl, "T":dbl, "Zbiornik 2":sgl})  [unwired: 1 in]
    n269 = Bundle("T"=w53, "T"=w55, "Zbiornik 3"=w10) -> (→"temp P5 - P6":cluster{"T":dbl, "T":dbl, "Zbiornik 3":sgl})  [unwired: 1 in]
    n270 = Divide(x=w7, y=sgl 3.0) -> (x/y=w9:sgl)
    n271 = Bundle("T"=w52, "T"=w54, w9) -> (→"temp P7 - P8":cluster{"T":dbl, "T":dbl, sgl})  [unwired: 1 in]
    n272 = local read "Zbiornik 4"() -> (w19:sgl)
    n273 = case shown="True" w117 {
      tunnel: w115 -> [_ w222]
      tunnel: [20.0 w221] -> w108
      tunnel: w109 -> [_ w220]
      tunnel: w110 -> [_ w219]
      tunnel: w111 -> [_ w218]
      tunnel: w112 -> [_ w217]
      tunnel: w113 -> [_ w216]
      tunnel: w114 -> [_ w215]
      tunnel: w19 -> [_ w214]
      frame False {
      }
      frame True {
        n274 = local read "Grzałka 4"() -> (w213:bool)
        n275 = case shown="False" w213 {
          tunnel: w222 -> [w227 w234]
          tunnel: [w228 w233] -> w221
          tunnel: w220 -> [w224 _]
          tunnel: w219 -> [_ w230]
          tunnel: w218 -> [w225 _]
          tunnel: w217 -> [w226 _]
          tunnel: w216 -> [_ w231]
          tunnel: w215 -> [_ w232]
          tunnel: w214 -> [w223 w229]
          frame False {
            # "ON/Off"
            n276 = formula code="T=To+(Tn-To)*(r4+r4d*L/300);"("r4"=w225, "r4d"=w226, "To"=w224, "L"=w223, "Tn"=w227) -> ("T"=w228:dbl)
          }
          frame True {
            # "grzałka On/Off"
            n277 = formula code="T=Tk+(Tn-Tk)*(r3+r3d*L/300);"("r3"=w231, "r3d"=w232, "L"=w229, "Tk"=w230, "Tn"=w234) -> ("T"=w233:dbl)
          }
        }
      }
    }
    n278 = Less?(x=w19, y=sgl 0.1) -> (x < y?=w73:bool)
    n279 = case shown="True" w73 {
      tunnel: [w300 20.0] -> w41
      tunnel: w108 -> [w300 _]
      frame False {
      }
      frame True {
      }
    }
    n280 = Divide(x=w19, y=sgl 3.0) -> (x/y=w18:sgl)
    n281 = Bundle(w18, "T"=w41) -> (→"Temp i objętość cieczy w zb 4":cluster{sgl, "T":dbl})  [unwired: 1 in]
    n282 = To Single Precision Float(number=w41) -> (single precision float=→"Temp. cieczy w zb 4":sgl)
    "Inf - poz przed zb2" <- w79
    "Inf - poz przed zb3" <- w23
    "Inf - poz przed zb1" <- w13
    "Inf - temp przed zb4" <- w25
  }
